vi "Parse Core.vi"(0 "Vector Path in":refnum<class "Vector Abstract Path.lvclass">, 5 "Config Row":string[](array[string]), 11 "error in (no error)":errorcluster) -> (4 "Vector Path out":refnum<class "Vector Abstract Path.lvclass">, 15 "error out":errorcluster)   [LabVIEW 2023, in "RFFixtureCharact.Public.lvlib" / "Vector Abstract Path.lvclass"]
uses:
  Vector Abstract Path.lvclass
  Common/Base Classes/Path/Path.lvclass
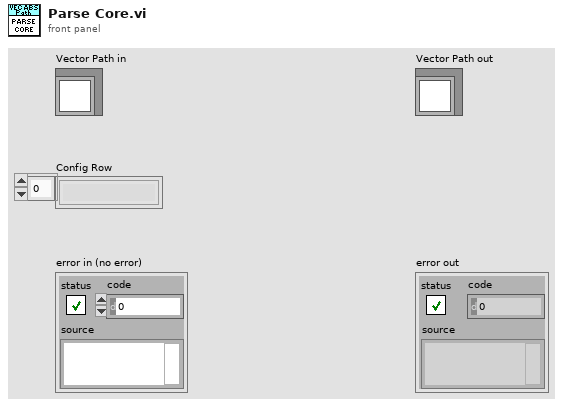
[diagram p1: front panel]
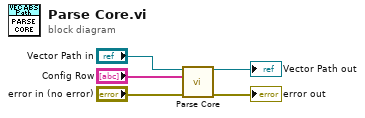
[diagram p0: block diagram]
diagram:
  n1 = call-parent "Parse Core.vi"("Path in"="Vector Path in", "Config Row"="Config Row", "error in (no error)"="error in (no error)") -> ("Path out"=→"Vector Path out":refnum<class "Vector Abstract Path.lvclass">, "error out"=→"error out":errorcluster)  [unwired: 11 in]
